vi "PMT_plus_Kiethley.vi"() -> ()   [LabVIEW 2022 SP3]
uses:
  <vilib>/Analysis/1siggen.llb/Ramp Pattern by Delta.vi
  <vilib>/Utility/file.llb/Write Delimited Spreadsheet (string).vi
  <vilib>/Utility/file.llb/Write Delimited Spreadsheet (DBL).vi
  <vilib>/Analysis/NI_AALBase.lvlib
  test_save_lv22/Close.vi/Close Folder/Users/Public/OneDrive/Desktop/Keithley_2450_2470_1_4_0_LV2015_NewReadme2_2450-LV2015-1.4.0/Keithley 2450/Keithley 2450.lvlib
panel:
  in  "Time to wait before current meas (ms)":i32
  in  "Use PMT?":bool=TRUE
  out "XY Graph":cluster{dbl[], dbl[]}(graph)
  out "Actual Voltage":dbl
  in  "Num Current Meas":i32=6
  in  "Path":path
  out "error out":errorcluster
  in  "error in (no error)":errorcluster
  in  "VISA resource name":refnum<visa-resource-name>
  out "Set Voltage":dbl
  in  "Step Size (V)":dbl=0.1 format="%#_13g"
  in  "Max V":dbl format="%#_13g"
  in  "Start V":dbl format="%#_13g"
  out "current":dbl
  in  "measurement interval":i32=200
  in  "Source Limit Level (0.1)":dbl=5e-08
  out "standard deviation":dbl
  out "mean":dbl
  out "data":u32[](array[numeric])
  out "OLD":bool
  out "DB":u32[](array[numeric])
  out "Overload":i32
  out "Gate Number":i32
  in  "Correction":bool=TRUE
  out "Num Gates Read":i32
  out "Gate Time Read":i32 caption="Gate time Read"
  out "Num Gates Set":i32=20
  out "Gate Time Set":i32=200
  out "PowerD":i32 caption="Power\nRead Data"
  out "Handle Number":i32
  # "as of now it only records every 1V"
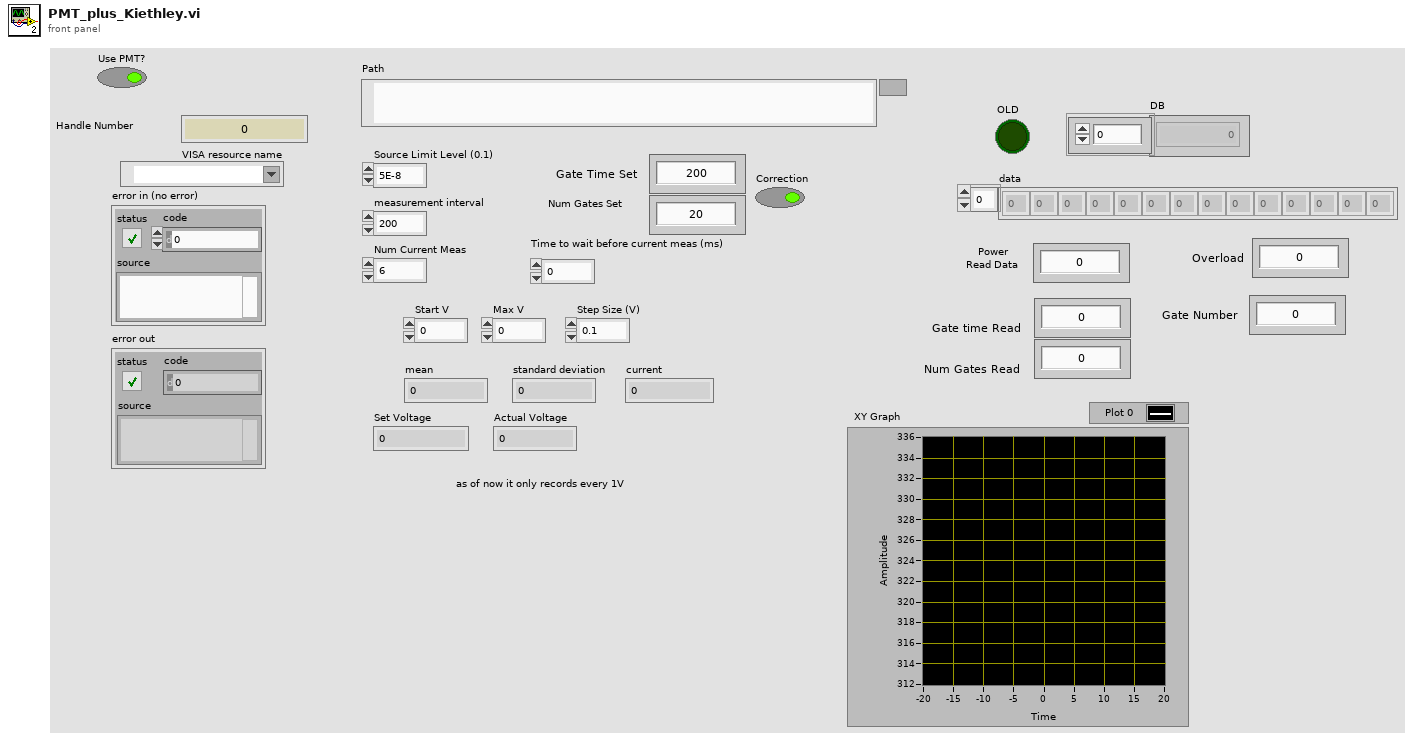
[diagram p1: front panel]
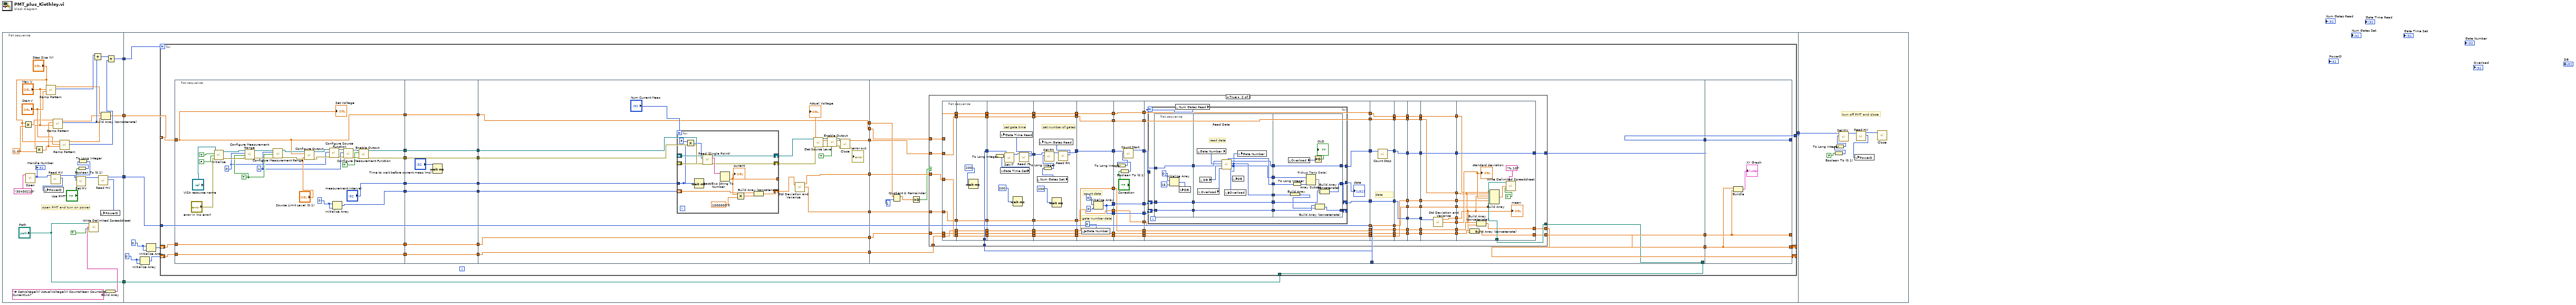
[diagram p0: block diagram]
diagram:
  n1 = flat-sequence {
    tunnel: [w25] -> w5
    tunnel: [w14] -> w4
    tunnel: [w13] -> w3
    tunnel: ["Path"] -> w1
    tunnel: w5 -> [w43]
    tunnel: w4 -> [w42]
    tunnel: w3 -> [w41]
    tunnel: [w40] -> w2
    tunnel: w1 -> [w39]
    tunnel: w2 -> [w437]
    frame #0 {
      w8 = -1.0
      # "open PMT and turn on power"
      n2 = Multiply(x="Step Size (V)", y=w8) -> (x*y=w6:dbl)
      n3 = call "Open.vi"("Serial Number"="30430219") -> ("Handle Number"=w29:i32)  [unwired: 9 in, 1 out]
      "Handle Number" <- w29
      n4 = Multiply(x="Max V", y=w8) -> (x*y=w16:dbl)
      n5 = call-poly <vilib>:"Ramp Pattern.vi"("start"="Start V", "end"="Max V", "delta"="Step Size (V)") -> ("samples"=w21:i32, "Ramp Pattern"=w18:dbl[])  [unwired: 6 in, 1 out]
      n6 = call "Read HV.vi"("handle"=w29) -> ("HV out"=w28:i32, "handle out"=w32:i32)  [unwired: 8 in, 1 out]
      n7 = local write "PowerD"(w28) -> ()
      n8 = call-poly <vilib>:"Ramp Pattern.vi"("start"="Max V", "end"=w16, "delta"=w6) -> ("samples"=w22:i32, "Ramp Pattern"=w19:dbl[])  [unwired: 6 in, 1 out]
      n9 = call-poly <vilib>:"Ramp Pattern.vi"("start"=w16, "end"="Start V", "delta"="Step Size (V)") -> ("samples"=w24:i32, "Ramp Pattern"=w20:dbl[])  [unwired: 6 in, 1 out]
      n10 = Boolean To (0,1)(Boolean="Use PMT?") -> (0, 1=w30:i16)
      n11 = To Long Integer(number=w30) -> (32bit integer=w31:i32)
      n12 = call "Set HV.vi"("HV"=w31, "handle"=w32) -> ("handle out"=w34:i32)  [unwired: 8 in, 1 out]
      n13 = Add(x=w21, y=w22) -> (x+y=w23:i32)
      n14 = call "Read HV.vi"("handle"=w34) -> ("HV out"=w33:i32, "handle out"=w25:i32)  [unwired: 8 in, 1 out]
      n15 = local write "PowerD"(w33) -> ()
      n16 = Build Array (concatenate)(w18, w19, w20) -> (w14:dbl[])
      n17 = Build Array("# SetVoltage(V) ActualVoltage(V) CountsMean CountsStd Current(uA)") -> (w10:string[])
      n18 = call-poly <vilib>:"Write Delimited Spreadsheet.vi"("file path (dialog if empty)"="Path", "1D data"=w10, "append to file? (new file:F)"=TRUE) -> ()  [unwired: 11 in, 2 out]
      n19 = Add(x=w23, y=w24) -> (x+y=w13:i32)
    }
    frame #1 {
      w37 = 0
      w38 = 0
      n20 = Initialize Array(w37, w37) -> (w36:i32[])
      n21 = Initialize Array(w38, w38) -> (w35:i32[])
      n22 = for {
        N: w41 -> [_]
        tunnel: w42 -> [w75] mode=indexing
        tunnel: w43 -> [w74]
        tunnel: [w73] -> w40
        tunnel: w39 -> [w72]
        shift-right: [w59] -> _
        shift-left: w35 -> [w67]
        shift-right: [w60] -> _
        shift-left: w36 -> [w66]
        n23 = flat-sequence {
          tunnel: w66 -> [w102]
          tunnel: w67 -> [w103]
          tunnel: w75 -> [w104]
          tunnel: [w104] -> w58
          tunnel: [w103] -> w56
          tunnel: [w102] -> w54
          tunnel: ["measurement interval"] -> w52
          tunnel: [w78] -> w50
          tunnel: [w77] -> w48
          tunnel: [w76] -> w46
          tunnel: w58 -> [w112]
          tunnel: [w112] -> w57
          tunnel: w56 -> [w111]
          tunnel: [w111] -> w55
          tunnel: w54 -> [w110]
          tunnel: [w110] -> w53
          tunnel: w52 -> [w109]
          tunnel: [w109] -> w51
          tunnel: w50 -> [w108]
          tunnel: [w108] -> w49
          tunnel: w48 -> [w107]
          tunnel: [w107] -> w47
          tunnel: w46 -> [w106]
          tunnel: [w106] -> w45
          tunnel: [w122] -> w71
          tunnel: [w123] -> w70
          tunnel: [w115] -> w69
          tunnel: [w122] -> w68
          tunnel: [w121] -> w65
          tunnel: [w120] -> w64
          tunnel: w57 -> [w122]
          tunnel: w55 -> [w121]
          tunnel: w53 -> [w120]
          tunnel: w51 -> [w119]
          tunnel: w49 -> [w118]
          tunnel: w47 -> [w117]
          tunnel: w45 -> [w116]
          tunnel: [w113] -> w44
          tunnel: w74 -> [w160]
          tunnel: w72 -> [w158]
          tunnel: w71 -> [w157]
          tunnel: w70 -> [w156]
          tunnel: w69 -> [w155]
          tunnel: w68 -> [w152]
          tunnel: w65 -> [w150]
          tunnel: w64 -> [w149]
          tunnel: [w159] -> w63
          tunnel: [w148] -> w62
          tunnel: [w147] -> w61
          tunnel: w44 -> [w146]
          tunnel: [w434] -> w59
          tunnel: [w435] -> w60
          tunnel: [w436] -> w73
          tunnel: w63 -> [w436]
          tunnel: w62 -> [w435]
          tunnel: w61 -> [w434]
          frame #0 {
            w86 = 0
            w85 = TRUE
            w82 = 1
            w84 = 0
            n24 = call "Initialize.vi"("error in (no error)"="error in (no error)", "Reset (True)"=FALSE, "ID Query (True)"=TRUE, "VISA resource name"="VISA resource name") -> ("error out"=w99:errorcluster, "VISA resource name out"=w100:refnum<visa-resource-name>)  [unwired: 6 in]
            n25 = call "Configure Measurement Range.vi"("error in (no error)"=w99, "Enable Auto Range (T:Enable)"=w85, "Function (0: Volts)"=w84, "VISA resource name"=w100) -> ("error out"=w98:errorcluster, "VISA resource name out"=w97:refnum<visa-resource-name>)  [unwired: 6 in]
            n26 = call "Configure Measurement Range.vi"("error in (no error)"=w98, "Enable Auto Range (T:Enable)"=w85, "Function (0: Volts)"=w82, "VISA resource name"=w97) -> ("error out"=w93:errorcluster, "VISA resource name out"=w89:refnum<visa-resource-name>)  [unwired: 6 in]
            n27 = call "Configure Output.vi"("VISA resource name"=w89, "Source Level (0)"=w104, "Source Limit Level (0.1)"="Source Limit Level (0.1)", "error in (no error)"=w93) -> ("VISA resource name out"=w90:refnum<visa-resource-name>, "error out"=w94:errorcluster)  [unwired: 10 in]
            n28 = call "Configure Source Function.vi"("error in (no error)"=w94, "Function (0: Volts)"=w84, "VISA resource name"=w90) -> ("error out"=w95:errorcluster, "VISA resource name out"=w91:refnum<visa-resource-name>)  [unwired: 7 in]
            n29 = Initialize Array(w86, w86) -> (w78:i32[])
            n30 = call "Configure Measurement Function.vi"("error in (no error)"=w95, "Function (0: Volts)"=w82, "VISA resource name"=w91) -> ("error out"=w96:errorcluster, "VISA resource name out"=w92:refnum<visa-resource-name>)  [unwired: 7 in]
            n31 = call "Enable Output.vi"("error in (no error)"=w96, "Enable Output (T: Enable)"=TRUE, "VISA resource name"=w92) -> ("error out"=w77:errorcluster, "VISA resource name out"=w76:refnum<visa-resource-name>)  [unwired: 7 in]
            "Set Voltage" <- w104
          }
          frame #1 {
            n32 = Wait (ms)(milliseconds to wait="Time to wait before current meas (ms)") -> ()  [unwired: 1 out]
          }
          frame #2 {
            n33 = for {
              N: "Num Current Meas" -> [_]
              tunnel: [w134] -> _
              shift-right: [w144] -> w129
              shift-left: w117 -> [w143]
              shift-right: [w142] -> w132
              shift-left: w116 -> [w141]
              tunnel: w119 -> [w138]
              shift-right: [w136] -> w114
              shift-left: w118 -> [w137]
              n34 = Multiply(x=3, y=w138) -> (x*y=w140:i32)
              n35 = Wait (ms)(milliseconds to wait=w138) -> ()  [unwired: 1 out]
              n36 = call "Read (Single Point).vi"("VISA resource name"=w141, "Timeout (10000 ms)"=w140, "error in (no error)"=w143) -> ("VISA resource name out"=w142:refnum<visa-resource-name>, "Data out"=w145:string, "error out"=w144:errorcluster)  [unwired: 10 in]
              n37 = Fract/Exp String To Number(string=w145) -> (number=w134:dbl)  [unwired: 3 in, 1 out]
              "current" <- w134
              n38 = Multiply(x=w134, y=1000000.0) -> (x*y=w133:dbl)
              n39 = Build Array (concatenate)(w137, w133) -> (w136:dbl[])
            }
            n40 = call <vilib>:"Std Deviation and Variance.vi"("X"=w114) -> ("mean"=w115:dbl, "standard deviation"=w113:dbl)  [unwired: 1 in, 1 out]
            n41 = call "Get Source Level.vi"("error in (no error)"=w129, "VISA resource name"=w132) -> ("error out"=w130:errorcluster, "Voltage Level Out"=w123:dbl, "VISA resource name out"=w131:refnum<visa-resource-name>)  [unwired: 6 in, 1 out]
            "Actual Voltage" <- w123
            n42 = call "Enable Output.vi"("error in (no error)"=w130, "Enable Output (T: Enable)"=TRUE, "VISA resource name"=w131) -> ("error out"=w125:errorcluster, "VISA resource name out"=w126:refnum<visa-resource-name>)  [unwired: 7 in]
            n43 = call "Close.vi"("error in (no error)"=w125, "VISA resource name"=w126) -> ("error out"=→"error out":errorcluster)  [unwired: 9 in]
          }
          frame #3 {
            n44 = Quotient & Remainder(x=w152, y=1) -> (x-y*floor(x/y)=w154:dbl)  [unwired: 1 out]
            n45 = Equal To 0?(x=w154) -> (x = 0?=w153:bool)
            n46 = case shown="True" w153 {
              tunnel: w160 -> [w163 w207]
              tunnel: [w163 w206] -> w159
              tunnel: w158 -> [_ w205]
              tunnel: w157 -> [_ w204]
              tunnel: w156 -> [_ w203]
              tunnel: w155 -> [_ w202]
              tunnel: w150 -> [w162 w201]
              tunnel: w149 -> [w161 w189]
              tunnel: [w162 w177] -> w148
              tunnel: [w161 w176] -> w147
              tunnel: w146 -> [_ w175]
              frame False {
              }
              frame True {
                n47 = flat-sequence {
                  tunnel: [w266] -> w260
                  tunnel: [w264] -> w259
                  tunnel: [w265] -> w258
                  tunnel: w204 -> [w266]
                  tunnel: w203 -> [w265]
                  tunnel: w202 -> [w264]
                  tunnel: w201 -> [w263]
                  tunnel: [w263] -> w190
                  tunnel: w189 -> [w262]
                  tunnel: [w262] -> w182
                  tunnel: w175 -> [w261]
                  tunnel: [w261] -> w171
                  tunnel: [w273] -> w257
                  tunnel: w207 -> [w273]
                  tunnel: [w272] -> w256
                  tunnel: w260 -> [w272]
                  tunnel: [w271] -> w255
                  tunnel: w259 -> [w271]
                  tunnel: [w270] -> w254
                  tunnel: w258 -> [w270]
                  tunnel: [w269] -> w191
                  tunnel: w190 -> [w269]
                  tunnel: [w268] -> w183
                  tunnel: w182 -> [w268]
                  tunnel: [w267] -> w172
                  tunnel: w171 -> [w267]
                  tunnel: w257 -> [w287]
                  tunnel: [w282] -> w253
                  tunnel: [w280] -> w252
                  tunnel: w256 -> [w280]
                  tunnel: [w279] -> w251
                  tunnel: w255 -> [w279]
                  tunnel: [w278] -> w250
                  tunnel: w254 -> [w278]
                  tunnel: [w277] -> w192
                  tunnel: w191 -> [w277]
                  tunnel: [w276] -> w184
                  tunnel: w183 -> [w276]
                  tunnel: [w275] -> w173
                  tunnel: w172 -> [w275]
                  tunnel: [w296] -> w249
                  tunnel: w253 -> [w298]
                  tunnel: [w293] -> w248
                  tunnel: w252 -> [w293]
                  tunnel: w251 -> [w292]
                  tunnel: [w292] -> w247
                  tunnel: [w291] -> w246
                  tunnel: w250 -> [w291]
                  tunnel: [w290] -> w193
                  tunnel: w192 -> [w290]
                  tunnel: [w289] -> w185
                  tunnel: w184 -> [w289]
                  tunnel: [w288] -> w174
                  tunnel: w173 -> [w288]
                  tunnel: w249 -> [w311]
                  tunnel: [w311] -> w245
                  tunnel: [w307] -> w244
                  tunnel: [w307] -> w243
                  tunnel: [w306] -> w242
                  tunnel: w248 -> [w306]
                  tunnel: [w305] -> w241
                  tunnel: w247 -> [w305]
                  tunnel: w246 -> [w304]
                  tunnel: [w304] -> w240
                  tunnel: [w303] -> w194
                  tunnel: w193 -> [w303]
                  tunnel: [w302] -> w186
                  tunnel: w185 -> [w302]
                  tunnel: w174 -> [w301]
                  tunnel: [w301] -> w167
                  tunnel: w245 -> [w324]
                  tunnel: [w320] -> w239
                  tunnel: w244 -> [w319]
                  tunnel: w243 -> [w318]
                  tunnel: [w319] -> w238
                  tunnel: [w318] -> w237
                  tunnel: w242 -> [w317]
                  tunnel: [w317] -> w236
                  tunnel: [w316] -> w235
                  tunnel: w241 -> [w316]
                  tunnel: [w315] -> w234
                  tunnel: w240 -> [w315]
                  tunnel: [w314] -> w195
                  tunnel: w194 -> [w314]
                  tunnel: [w313] -> w187
                  tunnel: w186 -> [w313]
                  tunnel: [w312] -> w168
                  tunnel: w167 -> [w312]
                  tunnel: [w337] -> w233
                  tunnel: w239 -> [w336]
                  tunnel: w238 -> [w335]
                  tunnel: w237 -> [w334]
                  tunnel: [w333] -> w232
                  tunnel: [w330] -> w231
                  tunnel: w236 -> [w330]
                  tunnel: [w329] -> w230
                  tunnel: w235 -> [w329]
                  tunnel: w234 -> [w328]
                  tunnel: [w328] -> w229
                  tunnel: [w327] -> w196
                  tunnel: w195 -> [w327]
                  tunnel: [w326] -> w188
                  tunnel: w187 -> [w326]
                  tunnel: [w325] -> w169
                  tunnel: w168 -> [w325]
                  tunnel: w233 -> [w391]
                  tunnel: [w390] -> w228
                  tunnel: [w389] -> w227
                  tunnel: w232 -> [w389]
                  tunnel: w231 -> [w388]
                  tunnel: [w388] -> w226
                  tunnel: [w387] -> w225
                  tunnel: w230 -> [w387]
                  tunnel: [w386] -> w224
                  tunnel: w229 -> [w386]
                  tunnel: [w385] -> w197
                  tunnel: w196 -> [w385]
                  tunnel: w188 -> [w384]
                  tunnel: [w384] -> w179
                  tunnel: [w383] -> w170
                  tunnel: w169 -> [w383]
                  tunnel: w228 -> [w398]
                  tunnel: w227 -> [w399]
                  tunnel: [w399] -> w223
                  tunnel: [w398] -> w222
                  tunnel: [w397] -> w221
                  tunnel: w226 -> [w397]
                  tunnel: w225 -> [w396]
                  tunnel: [w396] -> w220
                  tunnel: w224 -> [w395]
                  tunnel: [w395] -> w219
                  tunnel: [w394] -> w198
                  tunnel: w197 -> [w394]
                  tunnel: [w393] -> w180
                  tunnel: w179 -> [w393]
                  tunnel: w170 -> [w392]
                  tunnel: [w392] -> w164
                  tunnel: [w407] -> w218
                  tunnel: w223 -> [w407]
                  tunnel: [w406] -> w217
                  tunnel: w222 -> [w406]
                  tunnel: [w405] -> w216
                  tunnel: w221 -> [w405]
                  tunnel: [w404] -> w215
                  tunnel: w220 -> [w404]
                  tunnel: [w403] -> w214
                  tunnel: w219 -> [w403]
                  tunnel: [w402] -> w199
                  tunnel: w198 -> [w402]
                  tunnel: [w401] -> w181
                  tunnel: w180 -> [w401]
                  tunnel: [w400] -> w165
                  tunnel: w164 -> [w400]
                  tunnel: w218 -> [w417]
                  tunnel: [w416] -> w213
                  tunnel: [w415] -> w212
                  tunnel: [w414] -> w211
                  tunnel: w217 -> [w414]
                  tunnel: [w413] -> w210
                  tunnel: w216 -> [w413]
                  tunnel: [w412] -> w209
                  tunnel: w215 -> [w412]
                  tunnel: [w411] -> w208
                  tunnel: w214 -> [w411]
                  tunnel: [w410] -> w200
                  tunnel: w199 -> [w410]
                  tunnel: w181 -> [w409]
                  tunnel: [w409] -> w178
                  tunnel: [w408] -> w166
                  tunnel: w165 -> [w408]
                  tunnel: w213 -> [w422]
                  tunnel: w212 -> [w430]
                  tunnel: [w432] -> w206
                  tunnel: w211 -> [w432]
                  tunnel: w205 -> [w431]
                  tunnel: w210 -> [w425]
                  tunnel: w209 -> [w428]
                  tunnel: w208 -> [w421]
                  tunnel: w200 -> [w424]
                  tunnel: w178 -> [w423]
                  tunnel: [w420] -> w177
                  tunnel: [w419] -> w176
                  tunnel: w166 -> [w418]
                  frame #0 {
                  }
                  frame #1 {
                    n48 = Wait (ms)(milliseconds to wait=u32 200) -> ()  [unwired: 1 out]
                  }
                  frame #2 {
                    # "set gate time"
                    n49 = local read "Gate Time Set"() -> (w284:i32)
                    n50 = To Long Integer(number=w284) -> (32bit integer=w285:i32)
                    n51 = call "Set IT.vi"("IT"=w285, "handle"=w287) -> ("handle out"=w286:i32)  [unwired: 8 in, 1 out]
                    n52 = Wait (ms)(milliseconds to wait=u32 200) -> ()  [unwired: 1 out]
                    n53 = call "Read IT.vi"("handle"=w286) -> ("IT out"=w283:i32, "handle out"=w282:i32)  [unwired: 8 in, 1 out]
                    n54 = local write "Gate Time Read"(w283) -> ()
                  }
                  frame #3 {
                    # "set number of gates"
                    n55 = local read "Num Gates Set"() -> (w300:i32)
                    n56 = To Long Integer(number=w300) -> (32bit integer=w299:i32)
                    n57 = call "Set RN.vi"("RN"=w299, "handle"=w298) -> ("handle out"=w297:i32)  [unwired: 8 in, 1 out]
                    n58 = Wait (ms)(milliseconds to wait=u32 200) -> ()  [unwired: 1 out]
                    n59 = call "Read RN.vi"("handle"=w297) -> ("RN out"=w295:i32, "handle out"=w296:i32)  [unwired: 8 in, 1 out]
                    n60 = local write "Num Gates Read"(w295) -> ()
                  }
                  frame #4 {
                    # "gate number data"
                    # "count data"
                    n61 = local write "Gate Number"(0) -> ()
                    n62 = Initialize Array(u32 0, 0 ("次元サイズ")) -> (w307:u32[])
                  }
                  frame #5 {
                    n63 = Boolean To (0,1)(Boolean="Correction") -> (0, 1=w323:i16)
                    n64 = To Long Integer(number=w323) -> (32bit integer=w322:i32)
                    n65 = call "Count Start.vi"("Correction"=w322, "handle"=w324) -> ("handle out"=w320:i32)  [unwired: 8 in, 1 out]
                  }
                  frame #6 {
                    n66 = local read "Num Gates Read"() -> (w332:i32)
                    n67 = for {
                      N: w332 -> [_]
                      shift-right: [w338] -> w333
                      shift-left: w335 -> [w346]
                      shift-right: [w342] -> _
                      shift-left: w334 -> [w345]
                      tunnel: w336 -> [w347]
                      tunnel: [w348] -> w337
                      tunnel: [w338] -> w331
                      n68 = flat-sequence {
                        tunnel: [w358] -> w352
                        tunnel: [w357] -> w343
                        tunnel: [w356] -> w340
                        tunnel: w347 -> [w358]
                        tunnel: w346 -> [w357]
                        tunnel: w345 -> [w356]
                        tunnel: [w369] -> w351
                        tunnel: w352 -> [w368]
                        tunnel: [w363] -> w350
                        tunnel: [w362] -> w349
                        tunnel: [w361] -> w344
                        tunnel: w343 -> [w361]
                        tunnel: [w360] -> w341
                        tunnel: w340 -> [w360]
                        tunnel: [w359] -> w339
                        tunnel: w351 -> [w382]
                        tunnel: w350 -> [w377]
                        tunnel: w349 -> [w376]
                        tunnel: w344 -> [w374]
                        tunnel: w341 -> [w373]
                        tunnel: w339 -> [w372]
                        tunnel: [w382] -> w348
                        tunnel: [w375] -> w338
                        tunnel: [w370] -> w342
                        frame #0 {
                          n69 = Initialize Array(u32 0, 16 ("次元サイズ")) -> (w353:u32[])
                          n70 = local write "DB"(w353) -> ()
                        }
                        frame #1 {
                          # "read data"
                          n71 = local read "Gate Number"() -> (w367:i32)
                          n72 = local read "Overload"() -> (w366:i32)
                          n73 = local read "DB"() -> (w364:u32[])
                          n74 = call "Read Data.vi"("OLD"=w366, "DataBuf"=w364, "GateNum"=w367, "handle"=w368) -> ("OLD out"=w365:i32, "DataBuf out"=w362:u32[], "GateNum out"=w359:i32, "handle out"=w369:i32, "function return"=w363:u32)  [unwired: 3 in]
                          n75 = local write "Overload"(w365) -> ()
                          n76 = local write "DB"(w362) -> ()
                          n77 = local write "Gate Number"(w359) -> ()
                        }
                        frame #2 {
                          # "Pickup Tans Data!"
                          n78 = local read "Overload"() -> (w380:i32)
                          n79 = Build Array(w372) -> (w371:i32[])
                          n80 = To Long Integer(number=w377) -> (32bit integer=w378:i32)
                          n81 = Array Subset(array=w376, length=w378) -> (w379:u32[])  [unwired: 1 in]
                          n82 = Not Equal To 0?(x=w380) -> (x != 0?=→"OLD":bool)
                          n83 = Build Array (concatenate)(w373, w371) -> (w370:u32[])
                          n84 = Build Array (concatenate)(w374, w379) -> (w375:u32[])
                        }
                      }
                    }
                    "data" <- w331
                  }
                  frame #7 {
                    # "data"
                    n85 = call "Count Stop.vi"("handle"=w391) -> ("handle out"=w390:i32)  [unwired: 9 in, 1 out]
                  }
                  frame #8 {
                  }
                  frame #9 {
                  }
                  frame #10 {
                    n86 = call <vilib>:"Std Deviation and Variance.vi"("X"=w417) -> ("mean"=w416:dbl, "standard deviation"=w415:dbl)  [unwired: 1 in, 1 out]
                  }
                  frame #11 {
                    n87 = Build Array (concatenate)(w424, w422) -> (w419:dbl[])
                    n88 = Build Array (concatenate)(w423, w421) -> (w420:dbl[])
                    n89 = Build Array(w425, w421, w422, w430, w428, w418) -> (w429:dbl[])
                    n90 = call-poly <vilib>:"Write Delimited Spreadsheet.vi"("file path (dialog if empty)"=w431, "format (%.3f)"="%.10f", "1D data"=w429, "append to file? (new file:F)"=TRUE) -> ()  [unwired: 10 in, 2 out]
                    "mean" <- w422
                    "standard deviation" <- w430
                  }
                }
              }
            }
          }
          frame #4 {
            n91 = Bundle(w435, w434) -> (→"XY Graph":cluster{dbl[], dbl[]})  [unwired: 1 in]
          }
        }
      }
    }
    frame #2 {
      # "turn off PMT and close"
      n92 = Boolean To (0,1)(Boolean=FALSE) -> (0, 1=w442:i16)
      n93 = To Long Integer(number=w442) -> (32bit integer=w441:i32)
      n94 = call "Set HV.vi"("HV"=w441, "handle"=w437) -> ("handle out"=w439:i32)  [unwired: 8 in, 1 out]
      n95 = call "Read HV.vi"("handle"=w439) -> ("HV out"=w443:i32, "handle out"=w438:i32)  [unwired: 8 in, 1 out]
      n96 = local write "PowerD"(w443) -> ()
      n97 = call "Close.vi"("Handle"=w438) -> ()  [unwired: 9 in, 2 out]
    }
  }
